vi "231215_Spectrometer_Example_1.0.vi"() -> ()   [LabVIEW 2023]
doc: "Simple VI acquiring continously a spectrum, make the average of multiple acquisitions if needed.\nSome extras features are added such as saturation, color ramp display, etc."
uses:
  Utils/Status_Ctrl.ctl
  <instrlib>/Ocean Optics 2000 4000/Ocean Optics 2000 4000.lvlib
panel:
  out "Wavelength_Size":i32=3648
  in  "Tab Control":enum32{"Spectrometer", "Tools"}(tab)
  in  "Wavelength / Intensity limits":u16[][](array[numeric])=[[400, 750], [0, 2000]]
  in  "Intensity autoscale?":bool=TRUE
  in  "Averages":u8=1 min=1
  out "Spectrum":cluster{dbl[], dbl[]}(graph)
  in  "Status":T1=enum."Exit"
  in  "Integration time (s)":dbl=0.10000000000000003 min=0.001 max=10.0 step=0.1
  out "Color Ramp (zero is black)":u32[](array[colorbox])=[16711680, 11141375, 10879231, 10617087, 10289407, 10027263, 9765119, 9437439, 9175295, 8913151, 8651007, 8388863, 8061183, 7799039, 7536895, 7209215, 6947071, 6684927, 6422783, 6160639, 5832959, 5570815, 5308671, 4980991, 4718847, 4456703, 4194559, 3932415, 3604735, 3342591, 3080447, 2752767, 2490623, 2228479, 1966335, 1704191, 1376511, 1114367, 852223, 524543, 262399, 255, 1535, 2815, 4095, 5375, 6911, 8191, 9471, 10751, 12031, 13311, 14591, 15871, 17151, 18431, 19711, 21247, 22527, 23807, 25087, 26367, 27647, 28927, 30207, 31487, 33023, 34303, 35583, 36863, 38143, 39423, 40703, 41983, 43263, 44543, 45823, 47359, 48639, 49919, 51199, 52479, 53759, 55039, 56319, 57599, 59135, 60415, 61695, 62975, 64255, 65535, 65522, 65510, 65497, 65484, 65471, 65458, 65446, 65433, 65420, 65408, 65395, 65382, 65369, 65356, 65344, 65331, 65318, 65306, 65293, 65280, 327424, 524032, 786176, 1048320, 1244928, 1507072, 1769216, 1965824, 2227968, 2424576, 2686720, 2948864, 3145472, 3407616, 3669760, 3866368, 4128512, 4390656, 4587264, 4849408, 5046016, 5308160, 5570304, 5766912, 6029056, 6291200, 6487808, 6749952, 7012096, 7208704, 7470848, 7732992, 7929600, 8191744, 8453888, 8650496, 8912640, 9109248, 9371392, 9633536, 9830144, 10092288, 10354432, 10551040, 10813184, 11075328, 11271936, 11534080, 11730688, 11992832, 12254976, 12451584, 12713728, 12975872, 13172480, 13434624, 13696768, 13893376, 14155520, 14417664, 14614272, 14876416, 15138560, 15335168, 15597312, 15793920, 16056064, 16318208, 16514816, 16776960, 16775936, 16774912, 16773888, 16772864, 16771840, 16770816, 16770048, 16769024, 16768000, 16766976, 16765952, 16764928, 16763904, 16762880, 16761856, 16760832, 16759808, 16758784, 16757760, 16756992, 16755968, 16754944, 16753920, 16752896, 16751872, 16750848, 16749824, 16748800, 16747776, 16746752, 16745728, 16744704, 16743936, 16742912, 16741888, 16740864, 16739840, 16738816, 16737792, 16736768, 16735744, 16734720, 16733696, 16732672, 16731648, 16730880, 16729856, 16728832, 16727808, 16726784, 16725760, 16724736, 16723712, 16722688, 16721664, 16720640, 16719616, 16718592, 16717824, 16716800, 16715776, 16714752, 16713728, 16712704, 16711680, 16711680, 16711680, 16711680, 16711680, 16711680, 16711680, 16711680, 16711680, 16711680, 16711680, 16711680, 16711680, 16711680, 16711680, 16711680, 16711680, 16711680, 16711680, 16711680, 16711680, 16711680, 16711680, 16711680, 16711680, 16711680, 16711680, 16711680, 16711680, 16711680, 16711680, 16711680, 16711680, 16711680, 16711680, 16711680, 16711680, 16711680, 16711680, 16711680, 16711680, 16711680, 16711680, 16711680, 16711680, 16711680, 16711680, 16711680, 16711680, 16711680, 16711680, 16711680, 16711680, 16711680, 16711680, 16711680, 16711680, 16711680, 16711680, 16711680, 16711680, 16711680, 16711680, 16711680, 16711680, 16711680, 16711680, 16711680, 16711680, 16711680, 16711680, 16711680, 16711680, 16711680, 16711680, 16711680, 16711680, 16711680, 16711680, 16711680, 16711680, 16711680, 16711680, 16711680, 16711680, 16711680, 16711680, 16711680, 16711680, 16711680, 16711680, 16711680, 16711680, 16711680, 16711680, 16711680, 16711680, 16711680, 16711680, 16711680, 16711680, 16711680, 16711680, 16711680]
  out "error out":errorcluster
  in  "error in":errorcluster
  # "Programmed by Sébastien Mailfert"
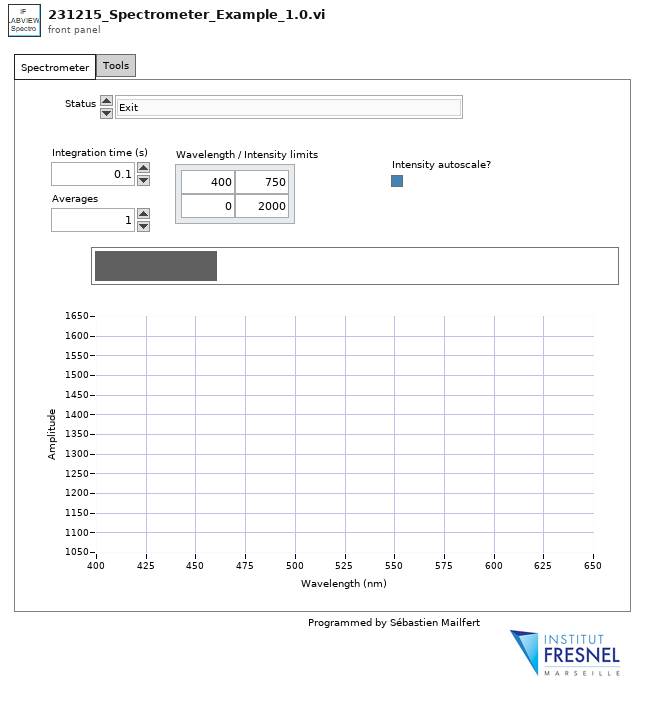
[diagram p1: front panel]
types:
  T1 = typedef "Status_Ctrl.ctl" = enum16{"Init", "Live", "Exit"}
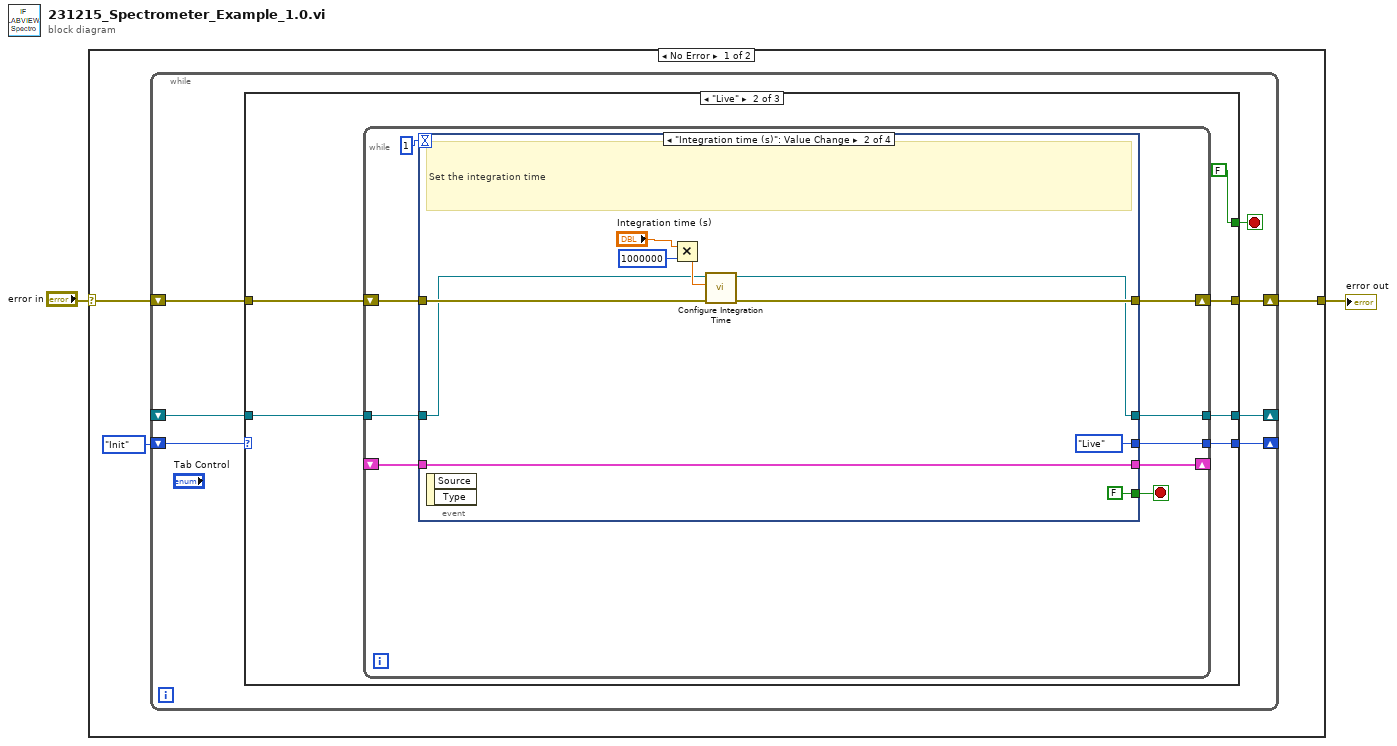
[diagram p0: block diagram]
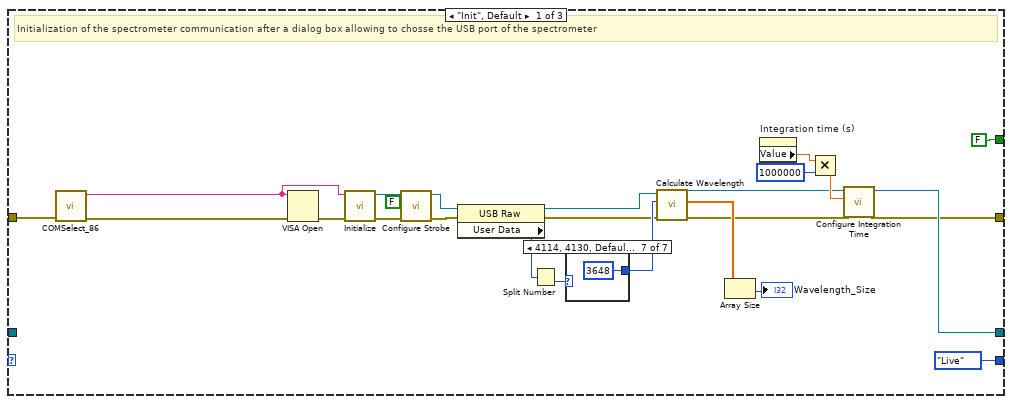
[diagram p2: hidden frame]
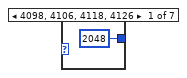
[diagram p3: hidden frame]
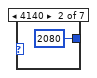
[diagram p4: hidden frame]
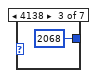
[diagram p5: hidden frame]
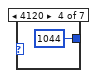
[diagram p6: hidden frame]
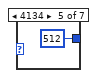
[diagram p7: hidden frame]
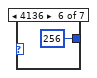
[diagram p8: hidden frame]
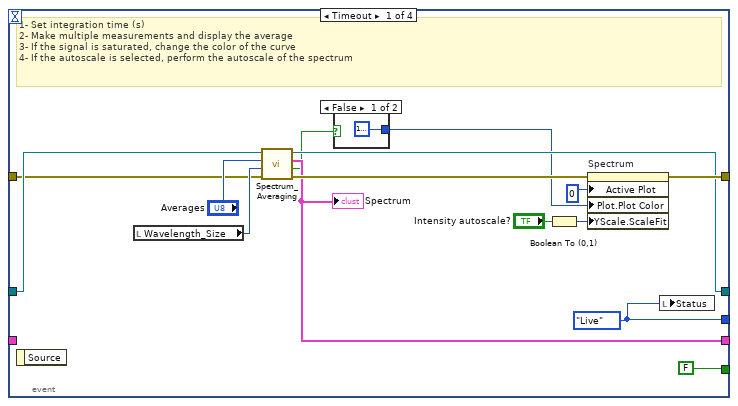
[diagram p9: hidden frame]
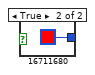
[diagram p10: hidden frame]
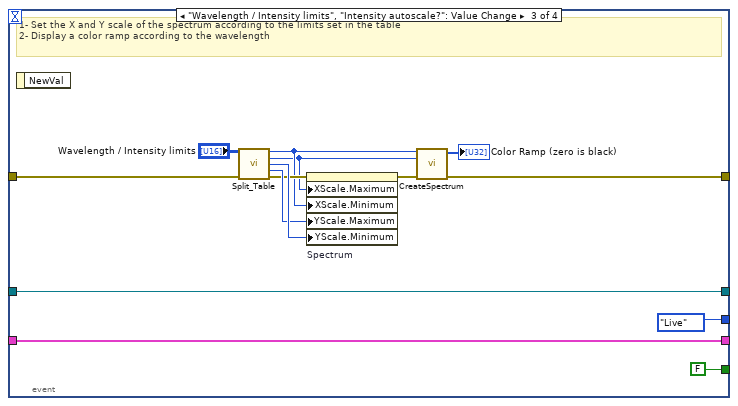
[diagram p11: hidden frame]
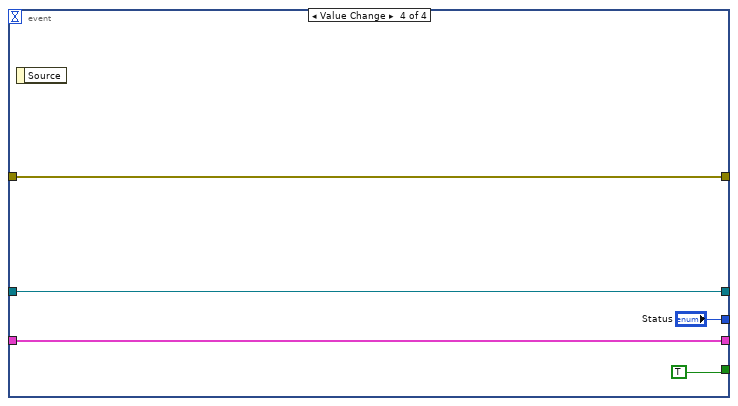
[diagram p12: hidden frame]
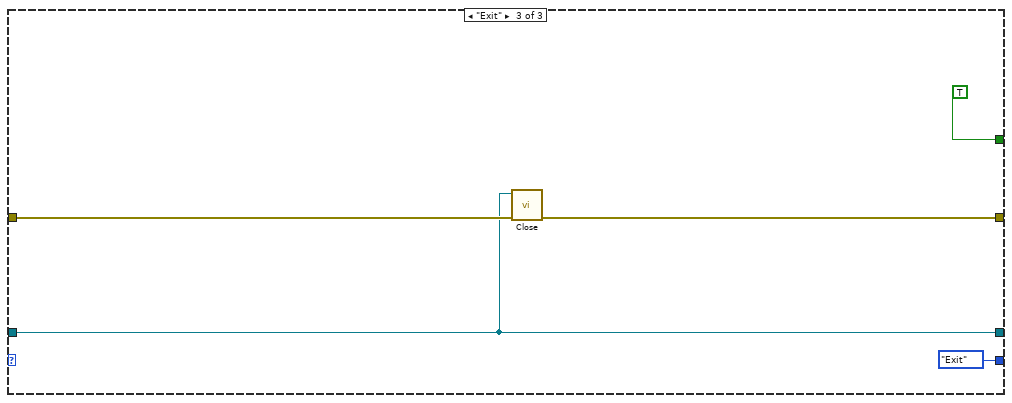
[diagram p13: hidden frame]
diagram:
  n1 = case shown="No Error" "error in" {
    selector: "error in" -> [w3 w111]
    tunnel: [w4 w111] -> w2
    frame No Error {
      n2 = while {
        shift-right: [w11] -> _
        shift-left: Status_Ctrl."Init" ("State") -> [w10]
        shift-right: [w9] -> w4
        shift-left: w3 -> [w8]
        shift-right: [w7] -> _
        shift-left: _ -> [w6]
        stop <- w12 stop-if-true
        n3 = case shown="\"Live\"" w10 {
          tunnel: [FALSE FALSE TRUE] -> w12
          tunnel: [Status_Ctrl."Live" ("State") w45 Status_Ctrl."Exit" ("State")] -> w11
          tunnel: [w13 w49 w107] -> w9
          tunnel: w8 -> [w34 w46 w108]
          tunnel: [w14 w48 w106] -> w7
          tunnel: w6 -> [_ w47 w106]
          frame "Init", Default {
            # "Initialization of the spectrometer communication after a dialog box allowing to chosse the USB port of the spectrometer"
            n4 = call "COMSelect_86.vi"("error in (no error)"=w34) -> ("error out"=w36:errorcluster, "COM Port Selected"=w37:string)  [unwired: 8 out]
            n5 = VISA Open(error in (no error)=w36, VISA resource name=w37) -> (error out=w22:errorcluster)  [unwired: 4 out]
            n6 = call <instrlib>:"Initialize.vi"("error in (no error)"=w22, "VISA resource name"=w37) -> ("error out"=w23:errorcluster, "VISA resource name out"=w25:refnum<visa-resource-name>)  [unwired: 8 in]
            n7 = call <instrlib>:"Configure Strobe.vi"("error in (no error)"=w23, "Enable Strobe (Disabled)"=FALSE, "VISA resource name"=w25) -> ("error out"=w26:errorcluster, "VISA resource name out"=w24:refnum<visa-resource-name>)  [unwired: 7 in]
            n8 = property class="USB Raw"(reference=w24, error in=w26) -> (reference out=w28:refnum<visa-resource-name>, error out=w27:errorcluster, "User Data"=w31:u32)
            n9 = Split Number(x=w31) -> (lo(x)=w30:u16)  [unwired: 1 out]
            n10 = case shown="4114, 4130, Default" w30 {
              tunnel: [2048 ("Number of Pixels (3840)") 2080 ("Number of Pixels (3840)") 2068 ("Number of Pixels (3840)") 1044 ("Number of Pixels (3840)") 512 ("Number of Pixels (3840)") 256 ("Number of Pixels (3840)") 3648 ("Number of Pixels (3840)")] -> w29
              frame 4098, 4106, 4118, 4126 {
              }
              frame 4140 {
              }
              frame 4138 {
              }
              frame 4120 {
              }
              frame 4134 {
              }
              frame 4136 {
              }
              frame 4114, 4130, Default {
              }
            }
            n11 = call <instrlib>:"Calculate Wavelength.vi"("error in (no error)"=w27, "Number of Pixels (3648)"=w29, "VISA resource name"=w28) -> ("error out"=w16:errorcluster, "Wavelength (nm)"=w21:dbl[], "VISA resource name out"=w15:refnum<visa-resource-name>)  [unwired: 6 in]
            n12 = Array Size(array=w21) -> (size(s)=→"Wavelength_Size":i32)
            n13 = property on="Integration time (s)" class="DigNum (strict)"() -> ("Value"=w17:dbl)  [unwired: 2 in, 2 out]
            n14 = Multiply(x=w17, y=u32 1000000) -> (x*y=w19:dbl)
            n15 = call <instrlib>:"Configure Integration Time.vi"("error in (no error)"=w16, "Integration Time (6000)"=w19, "VISA resource name"=w15) -> ("error out"=w13:errorcluster, "VISA resource name out"=w14:refnum<visa-resource-name>)  [unwired: 7 in]
          }
          frame "Live" {
            n16 = while {
              tunnel: [w58] -> w48
              tunnel: w47 -> [w57]
              shift-right: [w59] -> w49
              shift-left: w46 -> [w56]
              tunnel: [w53] -> w45
              shift-right: [w52] -> _
              shift-left: _ -> [w51]
              stop <- w54 stop-if-true
              n17 = event shown="[1] \"Integration time (s)\": Value Change" {
                selector: _ -> [_ _ _ _]
                dyn-events: _ -> [_ _ _ _]
                timeout: 1 -> [_ _ _ _]
                tunnel: [w70 w82 w94 w105] -> w59
                tunnel: [w69 w81 w100 w104] -> w58
                tunnel: w57 -> [w61 w80 w100 w104]
                tunnel: w56 -> [w60 w83 w90 w105]
                tunnel: [FALSE FALSE FALSE TRUE] -> w54
                tunnel: [w73 Status_Ctrl."Live" ("Status") Status_Ctrl."Live" ("State") "Status"] -> w53
                tunnel: [w64 w79 w97 w101] -> w52
                tunnel: w51 -> [_ w79 w97 w101]
                event Timeout {
                  w73 = Status_Ctrl."Live" ("State")
                  # "1- Set integration time (s)\n2- Make multiple measurements and display the average\n3- If the signal is saturated, change the color of the curve\n4- If the autoscale is selected, perform the autoscale of the spectrum"
                  n18 = event-data() -> ()  [unwired: 1 in, 1 out]
                  n19 = local read "Wavelength_Size"() -> (w63:i32)
                  n20 = call "Spectrum_Averaging.vi"("error in"=w60, "taille de la dimension"=w63, "Averages"="Averages", "VISA resource name in"=w61) -> ("error out"=w71:errorcluster, "Saturated?"=w62:bool, "XY Graph"=w64:cluster{dbl[], dbl[]}, "VISA resource name out"=w69:refnum<visa-resource-name>)  [unwired: 4 in]
                  "Spectrum" <- w64
                  n21 = case shown="False" w62 {
                    tunnel: [u32 16777224 u32 16711680] -> w68
                    frame False {
                    }
                    frame True {
                    }
                  }
                  n22 = Boolean To (0,1)(Boolean="Intensity autoscale?") -> (0, 1=w66:i16)
                  n23 = property on="Spectrum" class="XYGraph (strict)"(error in=w71, "Active Plot"=u32 0, "Plot.Plot Color"=w68, "YScale.ScaleFit"=w66) -> (error out=w70:errorcluster)  [unwired: 1 in, 1 out]
                  n24 = local write "Status"(w73) -> ()
                }
                event "Integration time (s)": Value Change {
                  # "Set the integration time"
                  n25 = event-data() -> ()  [unwired: 1 in, 2 out]
                  n26 = Multiply(x="Integration time (s)", y=u32 1000000) -> (x*y=w85:dbl)
                  n27 = call <instrlib>:"Configure Integration Time.vi"("error in (no error)"=w83, "Integration Time (6000)"=w85, "VISA resource name"=w80) -> ("error out"=w82:errorcluster, "VISA resource name out"=w81:refnum<visa-resource-name>)  [unwired: 7 in]
                }
                event "Wavelength / Intensity limits", "Intensity autoscale?": Value Change {
                  # "1- Set the X and Y scale of the spectrum according to the limits set in the table\n2- Display a color ramp according to the wavelength"
                  n28 = event-data() -> ()  [unwired: 1 in, 1 out]
                  n29 = call "Split_Table.vi"("Table (2x2) in"="Wavelength / Intensity limits", "error in"=w90) -> ("0,0"=w88:u16, "0,1"=w87:u16, "1,0"=w93:u16, "1,1"=w92:u16, "error out"=w91:errorcluster)  [unwired: 9 in]
                  n30 = property on="Spectrum" class="XYGraph (strict)"(error in=w91, "XScale.Maximum"=w87, "XScale.Minimum"=w88, "YScale.Maximum"=w92, "YScale.Minimum"=w93) -> (error out=w95:errorcluster)  [unwired: 1 in, 1 out]
                  n31 = call "CreateSpectrum.vi"("error in (no error)"=w95, "Lambda max"=w87, "Lambda min"=w88) -> ("error out"=w94:errorcluster, "Color Ramp (zero is black)"=→"Color Ramp (zero is black)":u32[])  [unwired: 7 in]
                }
                event Value Change {
                  n32 = event-data() -> ()  [unwired: 1 in, 1 out]
                }
              }
            }
          }
          frame "Exit" {
            n33 = call <instrlib>:"Close.vi"("error in (no error)"=w108, "VISA resource name"=w106) -> ("error out"=w107:errorcluster)  [unwired: 9 in]
          }
        }
      }
    }
    frame Error {
    }
  }
  "error out" <- w2
